vi "num channels in crate.vi"(2 "Crate Maps":T1(array[cluster]), 3 "crate":i32) -> (0 "Num channels in this crate":i32, 1 "Num channels in preceeding crates":i32)   [LabVIEW 2018]
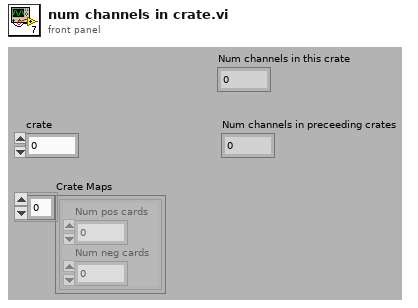
[diagram p1: front panel]
types:
  T1 = cluster{"Num pos cards":i32, "Num neg cards":i32}[]
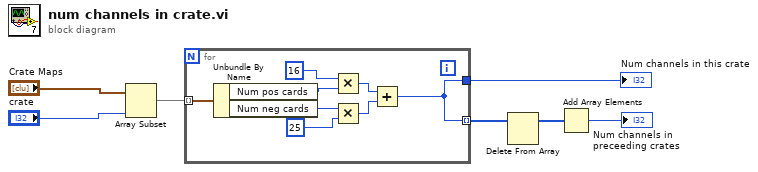
[diagram p0: block diagram]
diagram:
  n1 = Array Subset(array="Crate Maps", length="crate") -> (w7:T1)  [unwired: 1 in]
  n2 = for {
    tunnel: w7 -> [w15] mode=indexing
    tunnel: [w8] -> w2 mode=indexing
    tunnel: [w8] -> w4
    n3 = Unbundle By Name(w15) -> ("Num pos cards"=w14:i32, "Num neg cards"=w12:i32)
    n4 = Multiply(x=16, y=w14) -> (x*y=w10:i32)
    n5 = Multiply(x=w12, y=25 ("x")) -> (x*y=w9:i32)
    n6 = Add(x=w10, y=w9) -> (x+y=w8:i32)
  }
  "Num channels in this crate" <- w4
  n7 = Delete From Array(array=w2) -> (array with subset deleted=w1:i32[])  [unwired: 2 in, 1 out]
  n8 = Add Array Elements(numeric array=w1) -> (sum=→"Num channels in preceeding crates":i32)
